vi "DX3003_Setting.vi"(8 "ON/Off":bool, 9 "Voltage(V)":dbl, 10 "Current(mA)":dbl, 11 "Setup":string(combo)="VoltageOutput") -> (2 "Command":string)   [LabVIEW 2015]
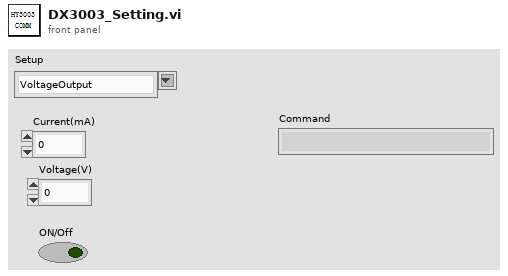
[diagram p1: front panel]
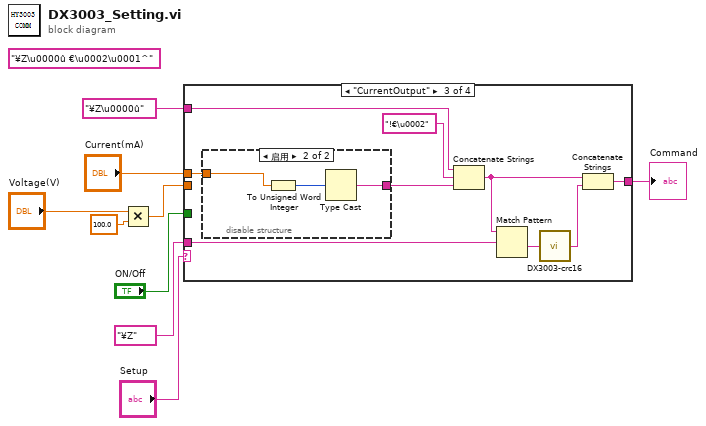
[diagram p0: block diagram]
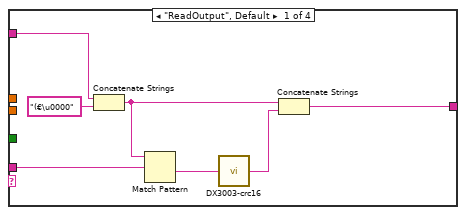
[diagram p2: hidden frame]
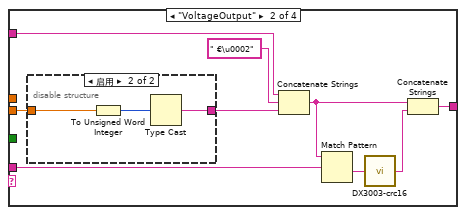
[diagram p3: hidden frame]
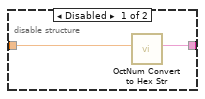
[diagram p4: hidden frame]
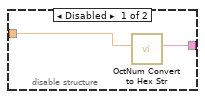
[diagram p5: hidden frame]
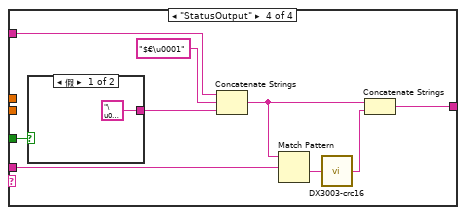
[diagram p6: hidden frame]
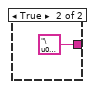
[diagram p7: hidden frame]
diagram:
  (unwired) "¥Z\u0000û €\u0002\u0001^" ("Write Command")
  n1 = Multiply(x="Voltage(V)", y=100.0) -> (x*y=w3:dbl)
  n2 = case shown="\"CurrentOutput\"" "Setup" {
    tunnel: "¥Z\u0000û" ("Write Command") -> [w13 w24 w38 w52]
    tunnel: w3 -> [_ w23 _ _]
    tunnel: "¥Z" ("Write Command") -> [w11 w21 w36 w51]
    tunnel: [w12 w18 w33 w48] -> w6
    tunnel: "Current(mA)" -> [_ _ w32 _]
    tunnel: "ON/Off" -> [_ _ _ w47]
    frame "ReadOutput", Default {
      n3 = Concatenate Strings(w13, "(€\u0000" ("Write Command")) -> (w14:string)
      n4 = Match Pattern(string=w14, regular expression=w11) -> (after substring=w10:string)  [unwired: 1 in, 3 out]
      n5 = call "DX3003-crc16.vi"("message"=w10) -> ("CRC16"=w15:string)  [unwired: 4 in]
      n6 = Concatenate Strings(w14, w15) -> (w12:string)
    }
    frame "VoltageOutput" {
      n7 = disable-structure shown="启用" {
        disable-tunnel: w23 -> [w27 w30]
        disable-tunnel: [w26 w28] -> w22
        frame Disabled {
          n8 = call "OctNum Convert to Hex Str.vi"("Voltage(V)"=w27) -> ("字符串"=w26:string)  [unwired: 10 in]
        }
        frame Enabled {
          n9 = To Unsigned Word Integer(number=w30) -> (unsigned 16bit integer=w29:u16)
          n10 = Type Cast(x=w29) -> (*(type *) &x=w28:string)  [unwired: 1 in]
        }
      }
      n11 = Concatenate Strings(w24, " €\u0002" ("Write Command"), w22) -> (w19:string)
      n12 = Match Pattern(string=w19, regular expression=w21) -> (after substring=w17:string)  [unwired: 1 in, 3 out]
      n13 = call "DX3003-crc16.vi"("message"=w17) -> ("CRC16"=w20:string)  [unwired: 4 in]
      n14 = Concatenate Strings(w19, w20) -> (w18:string)
    }
    frame "CurrentOutput" {
      n15 = disable-structure shown="启用" {
        disable-tunnel: [w41 w42] -> w37
        disable-tunnel: w32 -> [w40 w43]
        frame Disabled {
          n16 = call "OctNum Convert to Hex Str.vi"("Voltage(V)"=w40) -> ("字符串"=w41:string)  [unwired: 10 in]
        }
        frame Enabled {
          n17 = To Unsigned Word Integer(number=w43) -> (unsigned 16bit integer=w44:u16)
          n18 = Type Cast(x=w44) -> (*(type *) &x=w42:string)  [unwired: 1 in]
        }
      }
      n19 = Concatenate Strings(w38, "!€\u0002" ("Write Command"), w37) -> (w34:string)
      n20 = Match Pattern(string=w34, regular expression=w36) -> (after substring=w31:string)  [unwired: 1 in, 3 out]
      n21 = call "DX3003-crc16.vi"("message"=w31) -> ("CRC16"=w35:string)  [unwired: 4 in]
      n22 = Concatenate Strings(w34, w35) -> (w33:string)
    }
    frame "StatusOutput" {
      n23 = case shown="假" w47 {
        tunnel: ["\u0000" ("Write Command") "\u0001" ("Write Command")] -> w46
        frame False {
        }
        frame True {
        }
      }
      n24 = Concatenate Strings(w52, "$€\u0001" ("Write Command"), w46) -> (w49:string)
      n25 = Match Pattern(string=w49, regular expression=w51) -> (after substring=w45:string)  [unwired: 1 in, 3 out]
      n26 = call "DX3003-crc16.vi"("message"=w45) -> ("CRC16"=w50:string)  [unwired: 4 in]
      n27 = Concatenate Strings(w49, w50) -> (w48:string)
    }
  }
  "Command" <- w6
